vi "Set Waypoint type.vi"(8 "Error In":errorcluster, 11 "Waypoint Type In":T1) -> (0 "Error Out":errorcluster)   [LabVIEW 2014]
uses:
  Missions/Controls/Waypoint Type.ctl
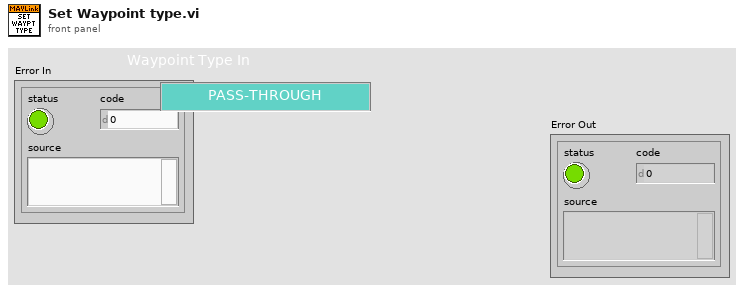
[diagram p1: front panel]
types:
  T1 = typedef "Waypoint Type.ctl" = enum16{"PASS-THROUGH", "INSPECT", "CIRCUMNAVIGATE"}
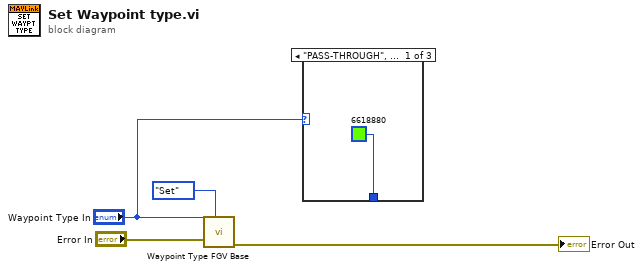
[diagram p0: block diagram]
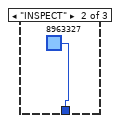
[diagram p2: hidden frame]
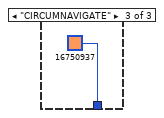
[diagram p3: hidden frame]
diagram:
  n1 = call "Waypoint Type FGV Base.vi"("Method"=enum16{"Get", "Set"}."Set", "Error In"="Error In", "Waypoint Type In"="Waypoint Type In") -> ("Error Out"=→"Error Out":errorcluster)  [unwired: 7 in, 1 out]
  n2 = case shown="\"PASS-THROUGH\", Default" "Waypoint Type In" {
    tunnel: [u32 6618880 u32 8963327 u32 16750937] -> _
    frame "PASS-THROUGH", Default {
    }
    frame "INSPECT" {
    }
    frame "CIRCUMNAVIGATE" {
    }
  }
